vi "FGV_PROXY_DIAGNOSTICS_message_history_buffer.vi"(6 "station":T2, 7 "options":T4, 8 "error_in":errorcluster, 11 "input":variant) -> (0 "error_out":errorcluster, 3 "message_history":T1[](array[typedef]))   [LabVIEW 2020]
uses:
  FGV_PROXY_DIAGNOSTICS_message_history_buffer.ctl
  STATION/station.ctl
  PROXY_DIAGNOSTICS_message_history_buffer_all_info.ctl
  _misc/DIAGNOSTICS_message_type.ctl
  main_ini/FGV_PROXY_config_info.ctl
  00c8a04a-a471-4d80-a66b-255c4561b6bb.vi
  6dde8c39-d05d-4c41-9577-428049675536.vi
  715657c1-86ea-4ea3-8139-0c93bcc0af77.vi
  edf3e8db-dbaf-4940-8721-95641f9dc414.vi
  dc9e6f03-6396-422b-a351-d5b3b188230c.vi
  <userlib>/_OpenG.lib/array/array.llb/Filter 1D Array with Scalar (Variant)__ogtk.vi
  <vilib>/addons/database/_DB Variant To Data/Database Variant To Data.xnode
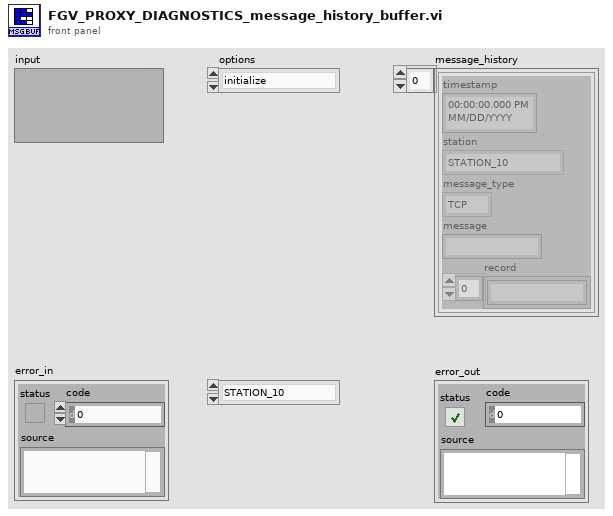
[diagram p1: front panel]
types:
  T1 = typedef "PROXY_DIAGNOSTICS_message_history_buffer_all_info.ctl" = cluster{"timestamp":timestamp, "station":T2, "message_type":T3, "message":string, "record":string[]}
  T2 = typedef "station.ctl" = enum16{"STATION_10", "STATION_20", "STATION_30", "STATION_40", "STATION_50", "STATION_60", "STATION_70", "STATION_80", "STATION_90", "STATION_100", "STATION_110", "STATION_120", "STATION_165", "MAIN"}
  T3 = typedef "DIAGNOSTICS_message_type.ctl" = enum16{"TCP", "SQL"}
  T4 = typedef "FGV_PROXY_DIAGNOSTICS_message_history_buffer.ctl" = enum16{"initialize", "add_TCP_PLC_to_PC", "add_TCP_PC_to_PLC", "add_SQL_PC_to_DB", "add_SQL_transaction", "add_SQL_DB_to_PC", "get_station", "get_all", "clear_station", "clear_all", "save_log"}
  T5 = typedef "FGV_PROXY_config_info.ctl" = enum16{"initialize", "set", "get"}
  T6 = enum16{"open", "replace", "create", "open or create", "replace or create", "replace or create with confirmation"}
  T7 = typedef "PROXY_all_config_info.ctl" = cluster{"main_ini_file":T8, "SQL Password":string, "queue_refnums":T9, "number_of_stations":i32}
  T8 = typedef "PROXY_main_ini_file.ctl" = cluster{"SQL Driver":string, "SQL Server":string, "SQL Database":string, "SQL UID":string, "Reference table":string, "Reference history":string, "Archivisation CFG table":string, "Archivisation CFG history":string, "User table":string, "User history":string, "default language":string, "REF CHG listener IP":string, "REF CHG listener port":u16, "ST 10 name":string, "ST 10 listener IP":string, "ST 10 listener port":u16, "ST 20 name":string, "ST 20 listener IP":string, "ST 20 listener port":u16, "ST 30 name":string, "ST 30 listener IP":string, "ST 30 listener port":u16, "ST 40 name":string, "ST 40 listener IP":string, "ST 40 listener port":u16, "ST 50 name":string, "ST 50 listener IP":string, "ST 50 listener port":u16, "ST 60 name":string, "ST 60 listener IP":string, "ST 60 listener port":u16, "ST 70 name":string, "ST 70 listener IP":string, "ST 70 listener port":u16, "ST 80 name":string, "ST 80 listener IP":string, "ST 80 listener port":u16, "ST 90 name":string, "ST 90 listener IP":string, "ST 90 listener port":u16, "ST 100 name":string, "ST 100 listener IP":string, "ST 100 listener port":u16, "ST 110 name":string, "ST 110 listener IP":string, "ST 110 listener port":u16, "ST 120 name":string, "ST 120 listener IP":string, "ST 120 listener port":u16, "ST 165 name":string, "ST 165 listener IP":string, "ST 165 listener port":u16}
  T9 = typedef "PROXY_queue_refnums.ctl" = cluster{"ST_10_queue":refnum<queue>, "ST_20_queue":refnum<queue>, "ST_30_queue":refnum<queue>, "ST_40_queue":refnum<queue>, "ST_50_queue":refnum<queue>, "ST_60_queue":refnum<queue>, "ST_70_queue":refnum<queue>, "ST_80_queue":refnum<queue>, "ST_90_queue":refnum<queue>, "ST_100_queue":refnum<queue>, "ST_110_queue":refnum<queue>, "ST_120_queue":refnum<queue>, "ST_165_queue":refnum<queue>}
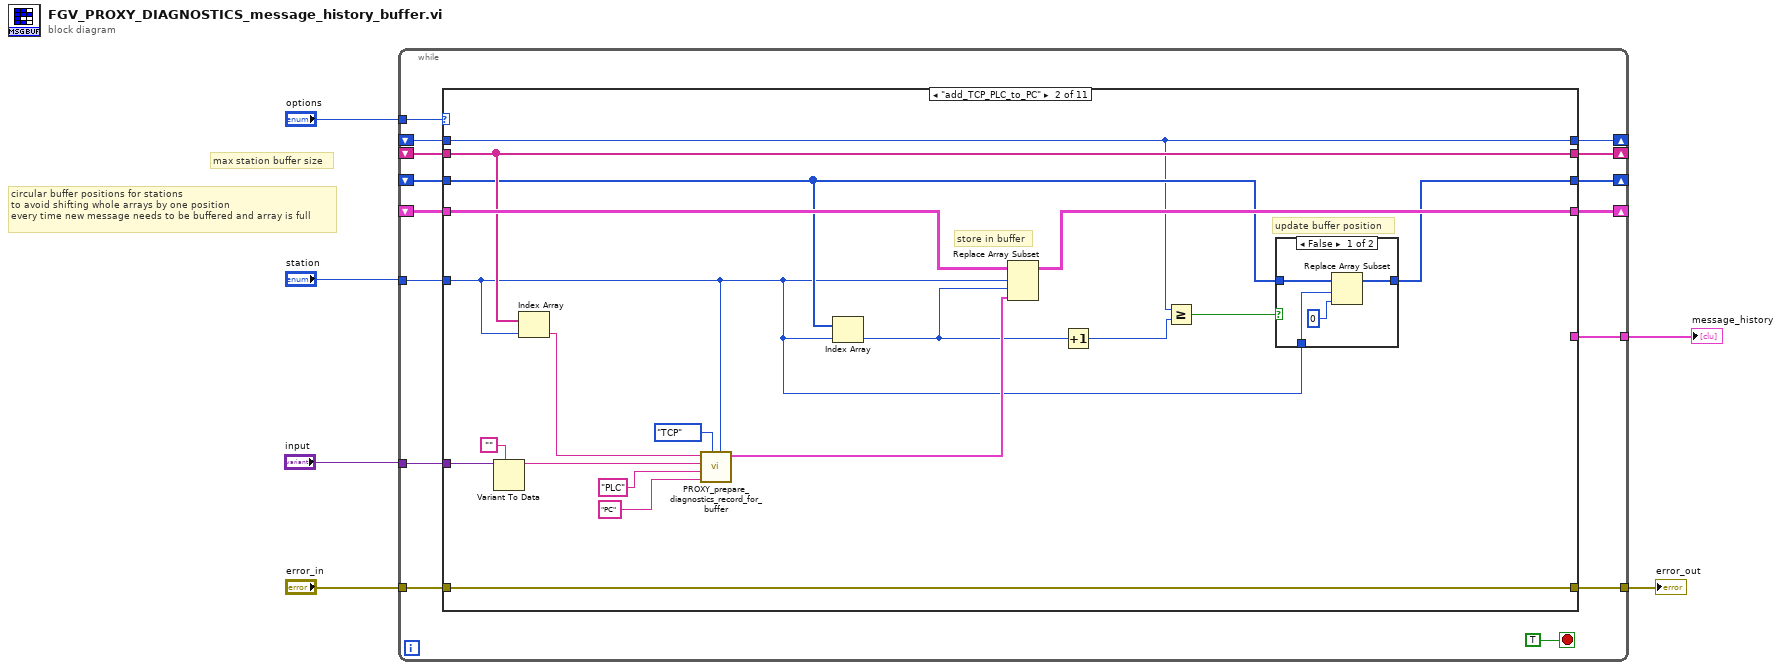
[diagram p0: block diagram]
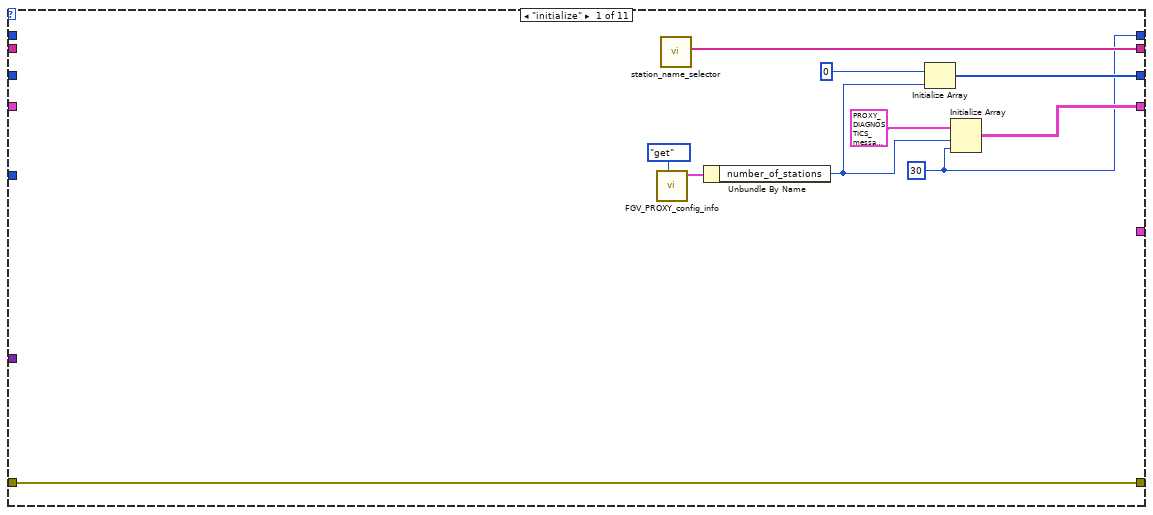
[diagram p2: hidden frame]
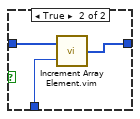
[diagram p3: hidden frame]
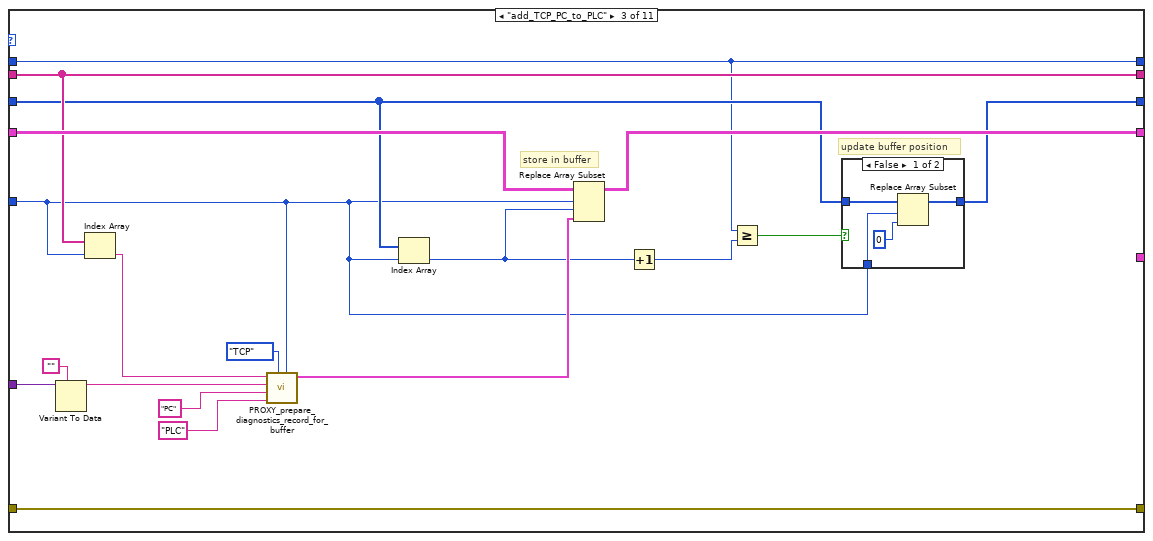
[diagram p4: hidden frame]
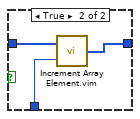
[diagram p5: hidden frame]
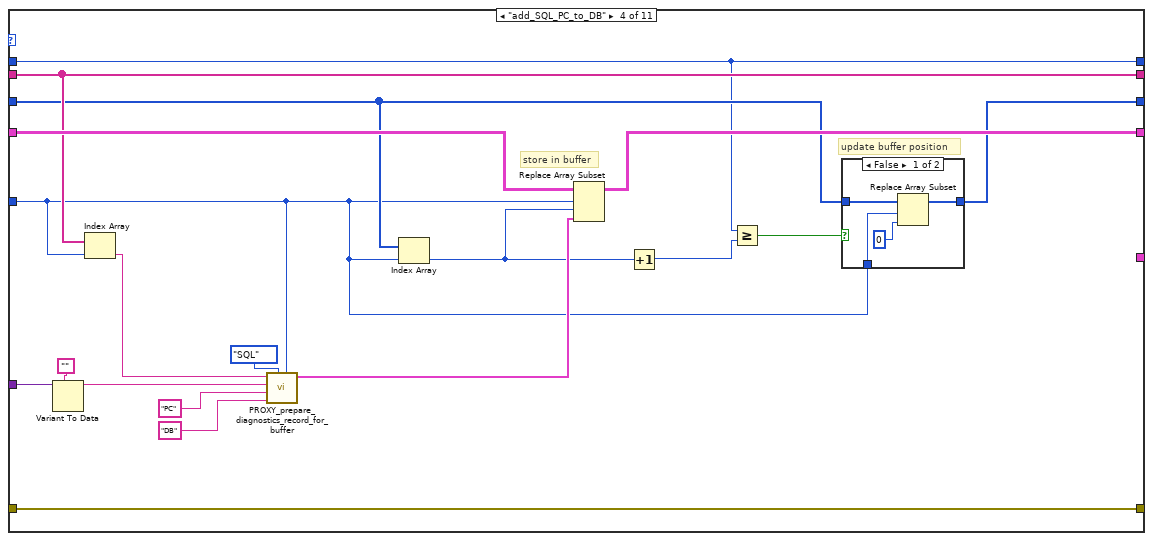
[diagram p6: hidden frame]
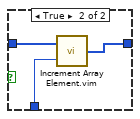
[diagram p7: hidden frame]
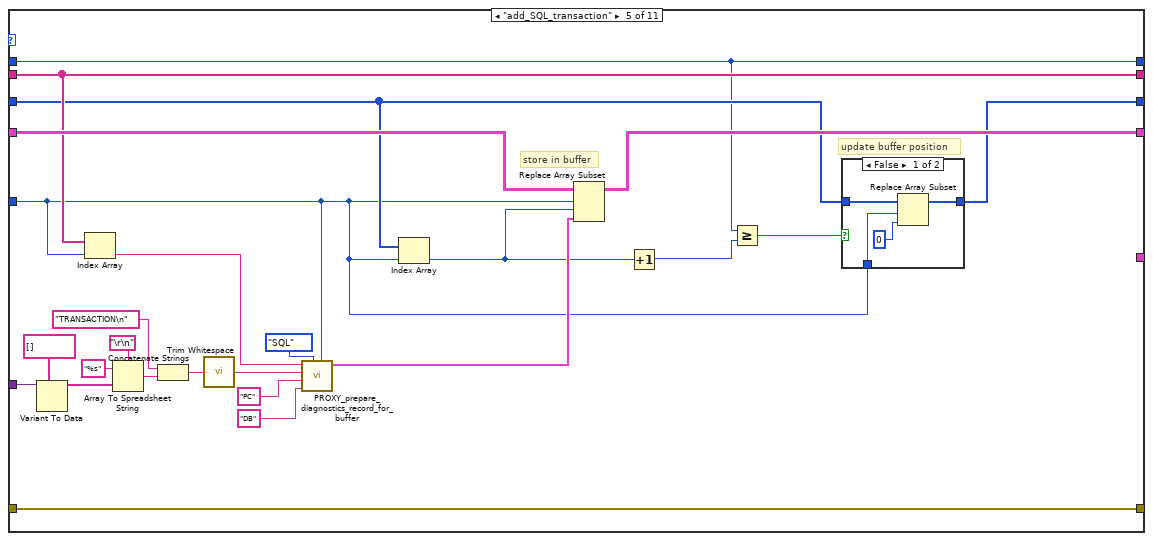
[diagram p8: hidden frame]
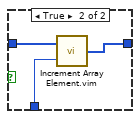
[diagram p9: hidden frame]
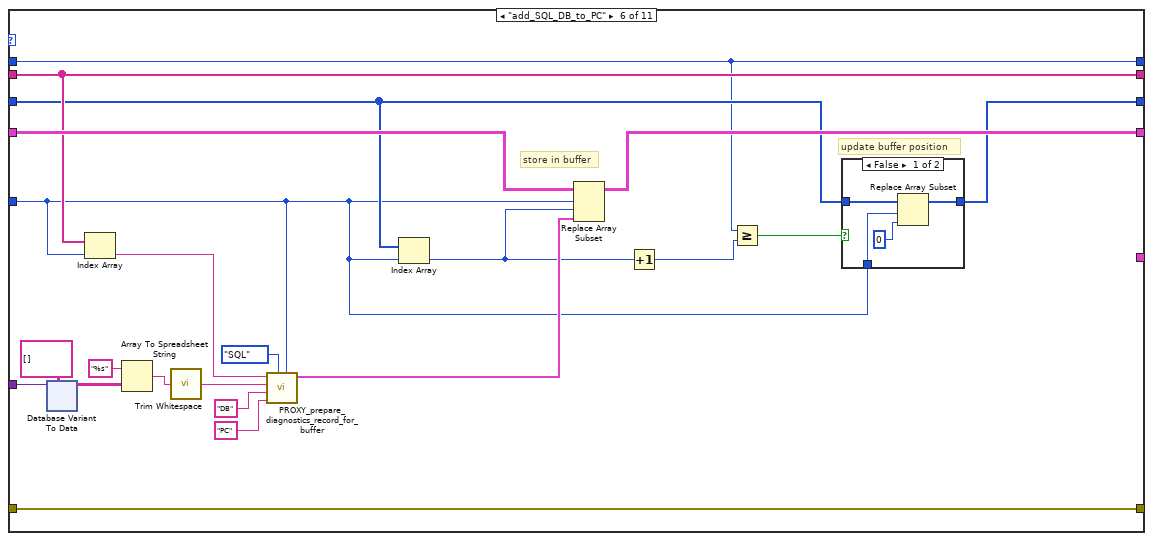
[diagram p10: hidden frame]
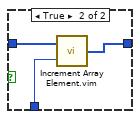
[diagram p11: hidden frame]
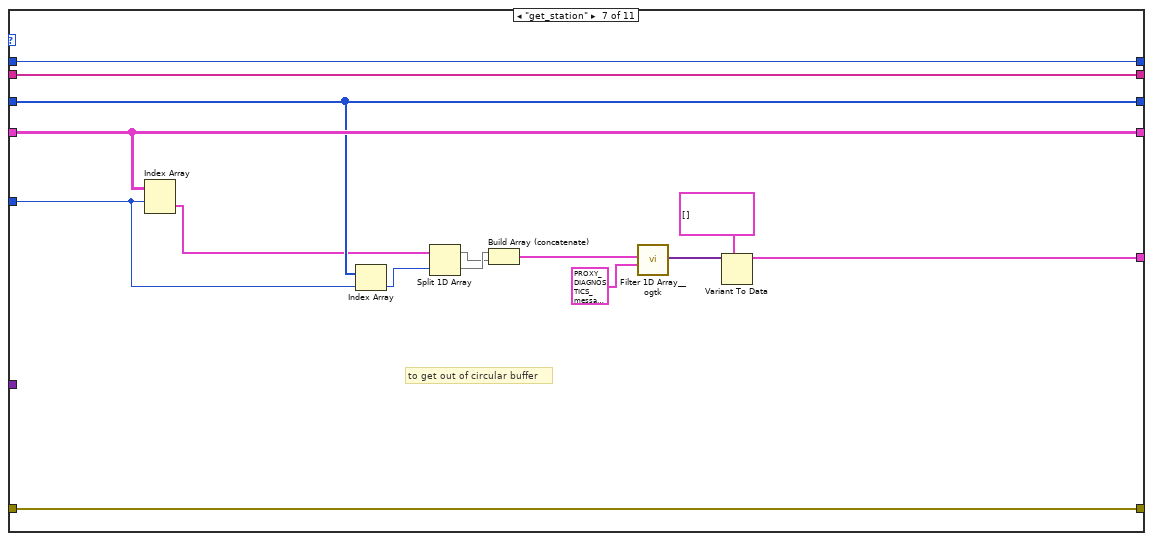
[diagram p12: hidden frame]
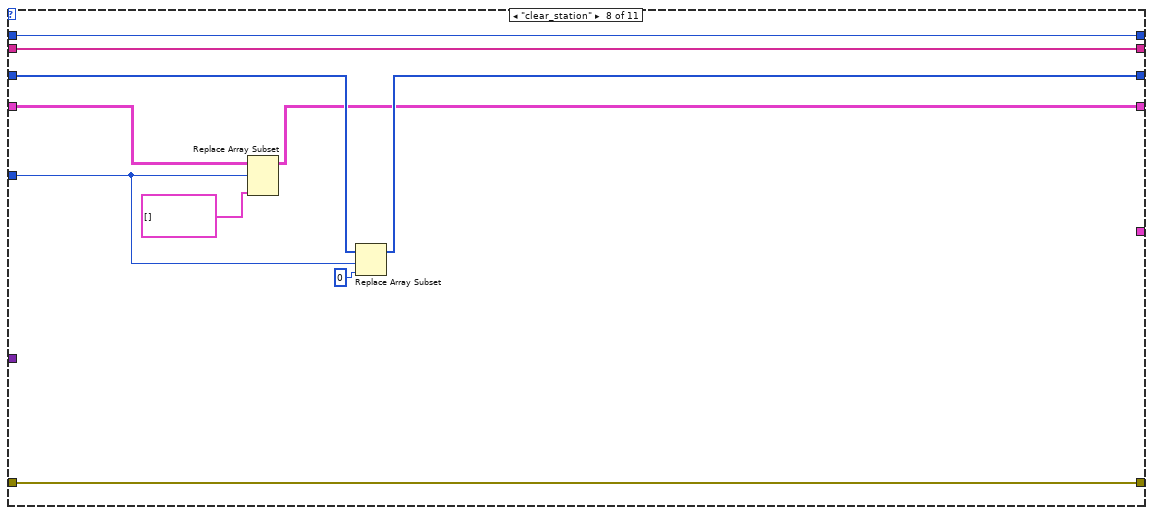
[diagram p13: hidden frame]
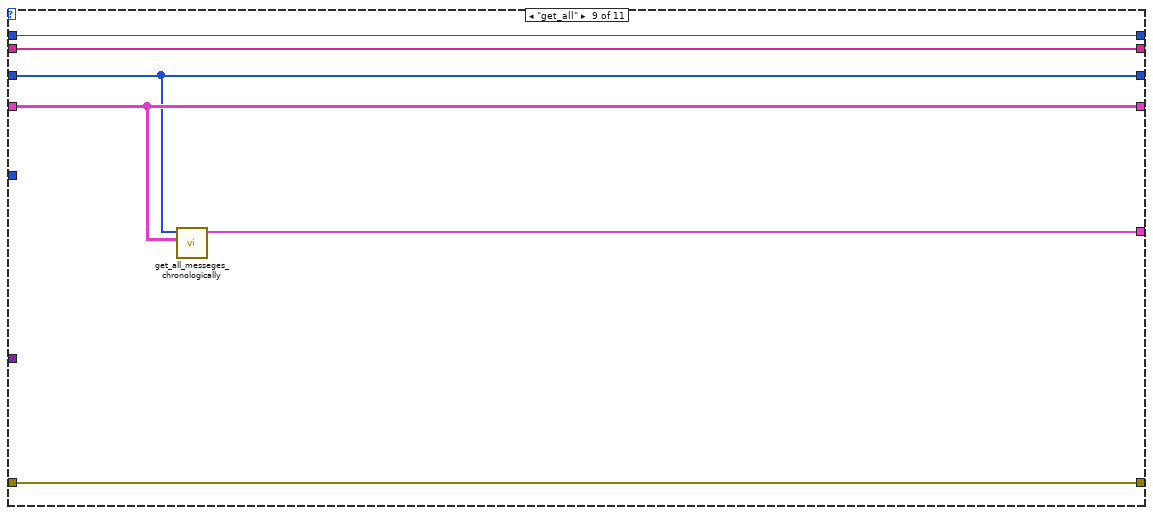
[diagram p14: hidden frame]
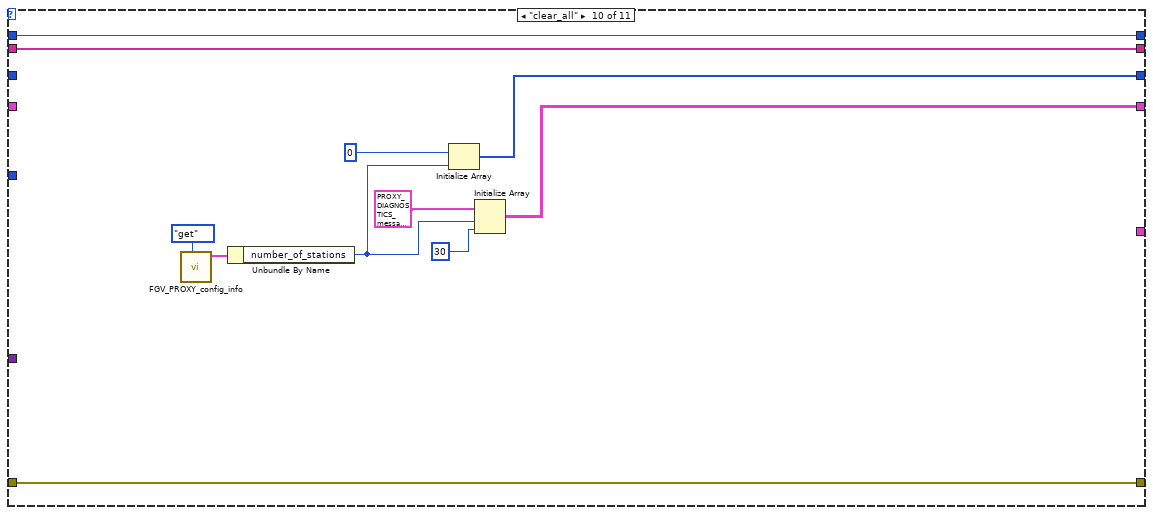
[diagram p15: hidden frame]
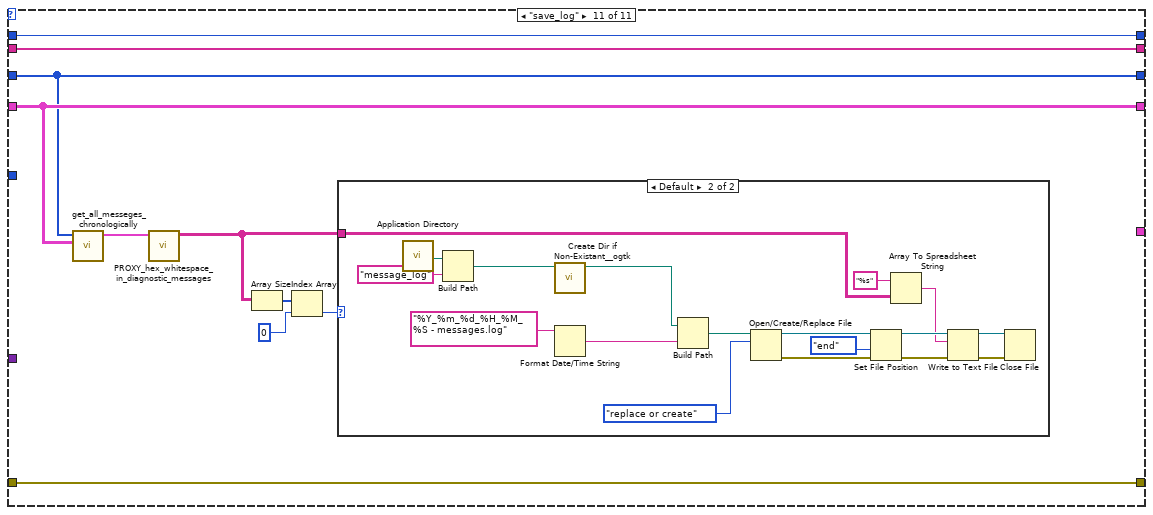
[diagram p16: hidden frame]
diagram:
  # "max station buffer size"
  # "circular buffer positions for stations\nto avoid shifting whole arrays by one position\nevery time new message needs to be buffered and array is full"
  n1 = while {
    tunnel: "options" -> [w20]
    tunnel: [w19] -> w6
    tunnel: "error_in" -> [w18]
    shift-right: [w17] -> _
    shift-left: _ -> [w15]
    tunnel: "station" -> [w16]
    tunnel: [w14] -> w2
    shift-right: [w13] -> _
    shift-left: _ -> [w12]
    tunnel: "input" -> [w11]
    shift-right: [w10] -> _
    shift-left: _ -> [w9]
    shift-right: [w8] -> _
    shift-left: _ -> [w7]
    stop <- TRUE stop-if-true
    n2 = case shown="\"add_TCP_PLC_to_PC\"" w20 {
      tunnel: [w31 w50 w76 w102 w134 w163 w217 w227 w233 w244 w254] -> w19
      tunnel: w18 -> [w31 w50 w76 w102 w134 w163 w217 w227 w233 w244 w254]
      tunnel: [w27 w42 w73 w99 w131 w160 w214 w218 w230 w234 w251] -> w17
      tunnel: w15 -> [_ w49 w75 w101 w133 w162 w214 w223 w230 _ w251]
      tunnel: w16 -> [_ w32 w58 w84 w118 w142 w212 w222 _ _ _]
      tunnel: [_ _ _ _ _ _ w203 _ w228 _ _] -> w14
      tunnel: [w26 w37 w71 w97 w129 w158 w213 w220 w229 w235 w250] -> w13
      tunnel: w12 -> [_ w38 w72 w98 w130 w159 w213 w224 w229 _ w250]
      tunnel: w11 -> [_ w35 w60 w86 w119 w147 _ _ _ _ _]
      tunnel: [w23 w47 w74 w100 w132 w161 w216 w226 w232 w243 w253] -> w10
      tunnel: w9 -> [_ w47 w74 w100 w132 w161 w216 w226 w232 w243 w253]
      tunnel: [w22 w36 w70 w96 w128 w157 w215 w225 w231 w242 w252] -> w8
      tunnel: w7 -> [_ w36 w70 w96 w128 w157 w215 w225 w231 w242 w252]
      frame "initialize" {
        w22 = 30 ("dimension size")
        n3 = call "FGV_PROXY_config_info.vi"("options"=FGV_PROXY_config_info."get") -> ("all_config_info_out"=w29:T7)  [unwired: 9 in, 1 out]
        n4 = call "station_name_selector.vi"() -> ("all_station_names"=w23:string[])  [unwired: 9 in, 2 out]
        n5 = Unbundle By Name(w29) -> ("number_of_stations"=w25:i32)
        n6 = Initialize Array(0, w25) -> (w26:i32[])
        n7 = Initialize Array(T1 {"timestamp"=timestamp(0 s since 1904-01-01), "station"=enum."STATION_10", "message_type"=enum."TCP", "message"="", "record"=[]} ("Cluster"), w25, w22) -> (w27:T1[][])
      }
      frame "add_TCP_PLC_to_PC" {
        # "update buffer position"
        # "store in buffer"
        n8 = Variant To Data(type="", Variant=w35) -> (data=w34:string)  [unwired: 1 in, 1 out]
        n9 = Index Array(array=w47, index=w32) -> (element=w46:string)
        n10 = call "PROXY_prepare_diagnostics_record_for_buffer.vi"("station"=w32, "message_type"=DIAGNOSTICS_message_type."TCP", "to"="PC" ("element"), "from"="PLC" ("element"), "message"=w34, "station_name"=w46) -> ("record"=w48:T1)  [unwired: 5 in]
        n11 = Index Array(array=w38, index=w32) -> (element=w41:i32)
        n12 = Replace Array Subset(array=w49, new element=w48, index (row)=w32, index (col)=w41) -> (w42:T1[][])
        n13 = Increment(x=w41) -> (x+1=w40:i32)
        n14 = Greater Or Equal?(x=w36, y=w40) -> (x >= y?=w39:bool)
        n15 = case shown="False" w39 {
          tunnel: w38 -> [w54 w57]
          tunnel: w32 -> [w53 w56]
          tunnel: [w51 w55] -> w37
          frame False {
            n16 = Replace Array Subset(array=w54, new element=0 ("new element/subarray"), index=w53) -> (w51:i32[])
          }
          frame True {
            n17 = call "Increment Array Element.vim"("index"=w56, "array in"=w57) -> ("array out"=w55:i32[])
          }
        }
      }
      frame "add_TCP_PC_to_PLC" {
        # "update buffer position"
        # "store in buffer"
        n18 = Variant To Data(type="", Variant=w60) -> (data=w59:string)  [unwired: 1 in, 1 out]
        n19 = Index Array(array=w74, index=w58) -> (element=w68:string)
        n20 = call "PROXY_prepare_diagnostics_record_for_buffer.vi"("station"=w58, "message_type"=DIAGNOSTICS_message_type."TCP", "to"="PLC" ("element"), "from"="PC" ("element"), "message"=w59, "station_name"=w68) -> ("record"=w69:T1)  [unwired: 5 in]
        n21 = Index Array(array=w72, index=w58) -> (element=w64:i32)
        n22 = Replace Array Subset(array=w75, new element=w69, index (row)=w58, index (col)=w64) -> (w73:T1[][])
        n23 = Increment(x=w64) -> (x+1=w63:i32)
        n24 = Greater Or Equal?(x=w70, y=w63) -> (x >= y?=w62:bool)
        n25 = case shown="False" w62 {
          tunnel: w72 -> [w80 w83]
          tunnel: w58 -> [w79 w82]
          tunnel: [w77 w81] -> w71
          frame False {
            n26 = Replace Array Subset(array=w80, new element=0 ("new element/subarray"), index=w79) -> (w77:i32[])
          }
          frame True {
            n27 = call "Increment Array Element.vim"("index"=w82, "array in"=w83) -> ("array out"=w81:i32[])
          }
        }
      }
      frame "add_SQL_PC_to_DB" {
        # "update buffer position"
        # "store in buffer"
        n28 = Variant To Data(type="", Variant=w86) -> (data=w85:string)  [unwired: 1 in, 1 out]
        n29 = Index Array(array=w100, index=w84) -> (element=w94:string)
        n30 = call "PROXY_prepare_diagnostics_record_for_buffer.vi"("station"=w84, "message_type"=DIAGNOSTICS_message_type."SQL", "to"="DB" ("element"), "from"="PC" ("element"), "message"=w85, "station_name"=w94) -> ("record"=w95:T1)  [unwired: 5 in]
        n31 = Index Array(array=w98, index=w84) -> (element=w90:i32)
        n32 = Replace Array Subset(array=w101, new element=w95, index (row)=w84, index (col)=w90) -> (w99:T1[][])
        n33 = Increment(x=w90) -> (x+1=w89:i32)
        n34 = Greater Or Equal?(x=w96, y=w89) -> (x >= y?=w88:bool)
        n35 = case shown="False" w88 {
          tunnel: w98 -> [w106 w109]
          tunnel: w84 -> [w105 w108]
          tunnel: [w103 w107] -> w97
          frame False {
            n36 = Replace Array Subset(array=w106, new element=0 ("new element/subarray"), index=w105) -> (w103:i32[])
          }
          frame True {
            n37 = call "Increment Array Element.vim"("index"=w108, "array in"=w109) -> ("array out"=w107:i32[])
          }
        }
      }
      frame "add_SQL_transaction" {
        # "update buffer position"
        # "store in buffer"
        n38 = Variant To Data(type=string[] [], Variant=w119) -> (data=w116:string[])  [unwired: 1 in, 1 out]
        n39 = Index Array(array=w132, index=w118) -> (element=w126:string)
        n40 = Array To Spreadsheet String(delimiter (Tab)="\r\n", array=w116, 3:"%s" ("format string")) -> (spreadsheet string=w113:string)
        n41 = Concatenate Strings("TRANSACTION\n" ("string"), w113) -> (w111:string)
        n42 = call <vilib>:"Trim Whitespace.vi"("string"=w111) -> ("trimmed string"=w110:string)  [unwired: 1 in]
        n43 = call "PROXY_prepare_diagnostics_record_for_buffer.vi"("station"=w118, "message_type"=DIAGNOSTICS_message_type."SQL", "to"="DB" ("element"), "from"="PC" ("element"), "message"=w110, "station_name"=w126) -> ("record"=w127:T1)  [unwired: 5 in]
        n44 = Index Array(array=w130, index=w118) -> (element=w122:i32)
        n45 = Replace Array Subset(array=w133, new element=w127, index (row)=w118, index (col)=w122) -> (w131:T1[][])
        n46 = Increment(x=w122) -> (x+1=w121:i32)
        n47 = Greater Or Equal?(x=w128, y=w121) -> (x >= y?=w120:bool)
        n48 = case shown="False" w120 {
          tunnel: w130 -> [w138 w141]
          tunnel: w118 -> [w137 w140]
          tunnel: [w135 w139] -> w129
          frame False {
            n49 = Replace Array Subset(array=w138, new element=0 ("new element/subarray"), index=w137) -> (w135:i32[])
          }
          frame True {
            n50 = call "Increment Array Element.vim"("index"=w140, "array in"=w141) -> ("array out"=w139:i32[])
          }
        }
      }
      frame "add_SQL_DB_to_PC" {
        # "update buffer position"
        # "store in buffer"
        n51 = xnode "Database Variant To Data"("database variant"=w147, "type"=string[][] []) -> ("data"=w146:string[][])  [unwired: 1 in, 1 out]
        n52 = Index Array(array=w161, index=w142) -> (element=w155:string)
        n53 = Array To Spreadsheet String(array=w146, 3:"%s" ("format string")) -> (spreadsheet string=w143:string)  [unwired: 1 in]
        n54 = call <vilib>:"Trim Whitespace.vi"("string"=w143) -> ("trimmed string"=w144:string)  [unwired: 1 in]
        n55 = call "PROXY_prepare_diagnostics_record_for_buffer.vi"("station"=w142, "message_type"=DIAGNOSTICS_message_type."SQL", "to"="PC" ("element"), "from"="DB" ("element"), "message"=w144, "station_name"=w155) -> ("record"=w156:T1)  [unwired: 5 in]
        n56 = Index Array(array=w159, index=w142) -> (element=w151:i32)
        n57 = Replace Array Subset(array=w162, new element=w156, index (row)=w142, index (col)=w151) -> (w160:T1[][])
        n58 = Increment(x=w151) -> (x+1=w150:i32)
        n59 = Greater Or Equal?(x=w157, y=w150) -> (x >= y?=w149:bool)
        n60 = case shown="False" w149 {
          tunnel: w159 -> [w199 w202]
          tunnel: w142 -> [w198 w201]
          tunnel: [w196 w200] -> w158
          frame False {
            n61 = Replace Array Subset(array=w199, new element=0 ("new element/subarray"), index=w198) -> (w196:i32[])
          }
          frame True {
            n62 = call "Increment Array Element.vim"("index"=w201, "array in"=w202) -> ("array out"=w200:i32[])
          }
        }
      }
      frame "get_station" {
        # "to get out of circular buffer"
        n63 = Index Array(array=w214, index (row)=w212) -> (element=w208:T1[])  [unwired: 1 in]
        n64 = Index Array(array=w213, index=w212) -> (element=w211:i32)
        n65 = Split 1D Array(array=w208, index=w211) -> (first subarray=w209:T1[], second subarray=w210:T1[])
        n66 = Build Array (concatenate)(w210, w209) -> (w207:T1[])
        n67 = call-poly <userlib>:"Filter 1D Array__ogtk.vi"("items to filter"=T1 {"timestamp"=timestamp(0 s since 1904-01-01), "station"=enum."STATION_10", "message_type"=enum."TCP", "message"="", "record"=[]} ("Cluster"), "array"=w207) -> ("filtered array"=w205:variant[])  [unwired: 4 in, 1 out]
        n68 = Variant To Data(type=T1[] [], Variant=w205) -> (data=w203:T1[])  [unwired: 1 in, 1 out]
      }
      frame "clear_station" {
        n69 = Replace Array Subset(array=w223, new element=T1[] [], index (row)=w222) -> (w218:T1[][])  [unwired: 1 in]
        n70 = Replace Array Subset(array=w224, new element=0 ("new element/subarray"), index=w222) -> (w220:i32[])
      }
      frame "get_all" {
        n71 = call "get_all_messeges_chronologically.vi"("DIAGNOSTIC_buffer_all_info"=w230, "circular_buffer_positions"=w229) -> ("all_messages"=w228:T1[])  [unwired: 9 in]
      }
      frame "clear_all" {
        n72 = call "FGV_PROXY_config_info.vi"("options"=FGV_PROXY_config_info."get") -> ("all_config_info_out"=w240:T7)  [unwired: 9 in, 1 out]
        n73 = Unbundle By Name(w240) -> ("number_of_stations"=w238:i32)
        n74 = Initialize Array(0, w238) -> (w235:i32[])
        n75 = Initialize Array(T1 {"timestamp"=timestamp(0 s since 1904-01-01), "station"=enum."STATION_10", "message_type"=enum."TCP", "message"="", "record"=[]} ("Cluster"), w238, 30 ("dimension size")) -> (w234:T1[][])
      }
      frame "save_log" {
        n76 = call "get_all_messeges_chronologically.vi"("DIAGNOSTIC_buffer_all_info"=w251, "circular_buffer_positions"=w250) -> ("all_messages"=w246:T1[])  [unwired: 9 in]
        n77 = call "PROXY_hex_whitespace_in_diagnostic_messages.vi"("message_history"=w246) -> ("hexed_records"=w245:string[][])  [unwired: 10 in]
        n78 = Array Size(array=w245) -> (size(s)=w249:i32[])
        n79 = Index Array(array=w249, index=0) -> (element=w247:i32)
        n80 = case shown="Default" w247 {
          tunnel: w245 -> [_ w272]
          frame 0 {
          }
          frame Default {
            n81 = call <vilib>:"Application Directory.vi"() -> ("Application Directory"=w258:path)
            n82 = Build Path(base path=w258, name or relative path="message_log") -> (appended path=w256:path)
            n83 = call <userlib>:"Create Dir if Non-Existant__ogtk.vi"("Directory Path"=w256) -> ("dup Directory Path"=w255:path)  [unwired: 8 in, 2 out]
            n84 = Format Date/Time String(time format string (%c)="%Y_%m_%d_%H_%M_%S - messages.log") -> (date/time string=w259:string)  [unwired: 2 in]
            n85 = Build Path(base path=w255, name or relative path=w259) -> (appended path=w264:path)
            n86 = Open/Create/Replace File(file path (use dialog)=w264, operation (0:open)=T6."replace or create") -> (refnum out=w268:refnum<file>, error out=w265:errorcluster)  [unwired: 4 in, 1 out]
            n87 = Set File Position(refnum=w268, from (0:start)=enum16{"start", "end", "current"}."end", error in=w265) -> (refnum out=w270:refnum<file>, error out=w266:errorcluster)  [unwired: 1 in]
            n88 = Array To Spreadsheet String(array=w272, 3:"%s" ("format string")) -> (spreadsheet string=w261:string)  [unwired: 1 in]
            n89 = Write to Text File(file (use dialog)=w270, text=w261, error in=w266) -> (refnum out=w263:refnum<file>, error out=w262:errorcluster)  [unwired: 1 in, 1 out]
            n90 = Close File(refnum=w263, error in=w262) -> ()  [unwired: 2 out]
          }
        }
      }
    }
  }
  "error_out" <- w6
  "message_history" <- w2
